vi "Test MultiValue INSERT.vi"() -> ()   [LabVIEW 2013, in "PQ Connection.lvclass"]
uses:
  Connection/PQ Connection.lvclass
  Result/PQ Result.lvclass/PQ Result.ctl
  Connection/Execute Command (No results).vi
  Result/Clear.vi
  Connection/Execute Command (Result).vi
  Connection/Execute (no results).vi
  Connection/Execute (Return first result with rows).vi
  Connection/Single Command with parameters.vi
  1. Sources/Lib/Lib.llb/Trim Whitespace (String)__ogtk.vi
panel:
  in  "Old":bool
  out "concatenated string":string
  in  "Connection Strings to access PostgreSQL":string="host=localhost port=5432 dbname = mydb "
  out "INSERTS/sec":dbl format="%#_3p"
  out "Time per INSERT":dbl format="%#_3p"
  out "error out":errorcluster
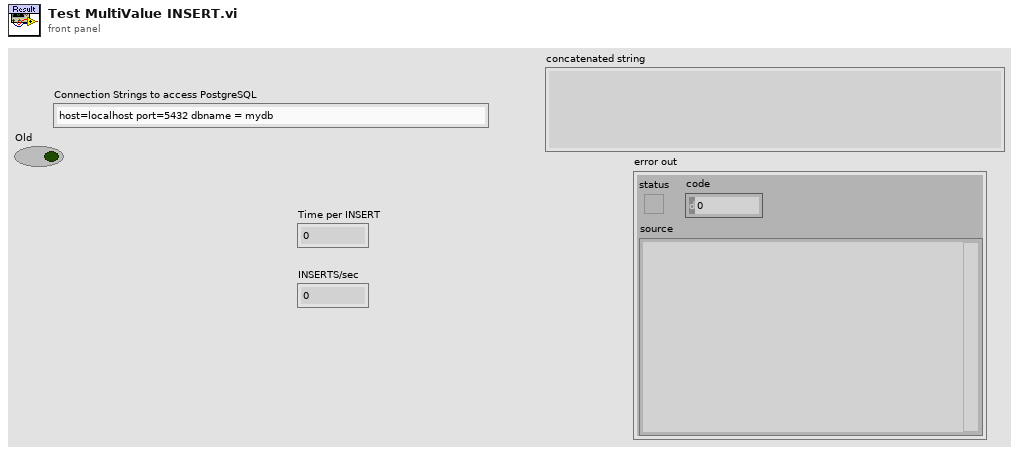
[diagram p1: front panel]
types:
  T1 = cluster{i32, "number: 0 to 1":dbl, string, "seconds since 1Jan1904":timestamp}
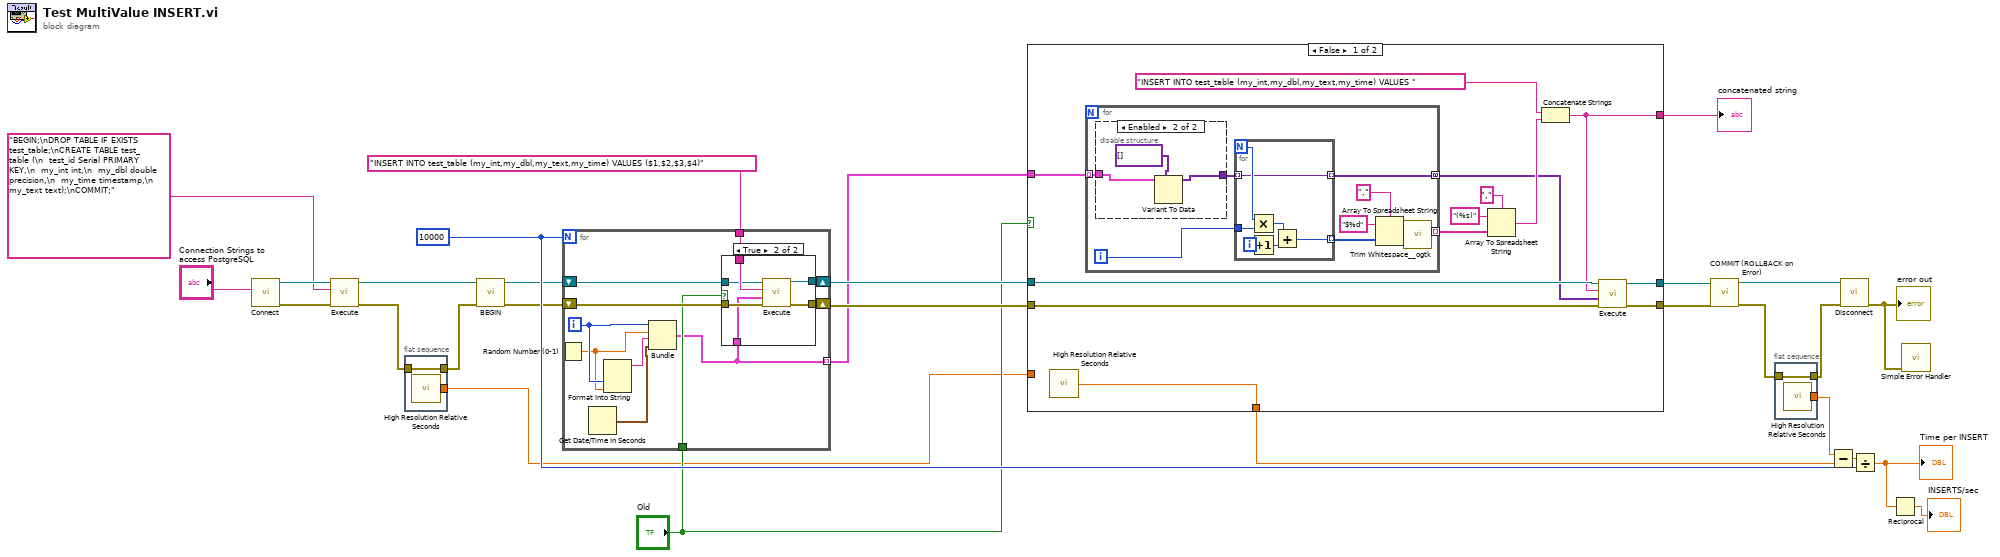
[diagram p0: block diagram]
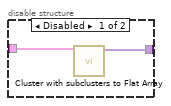
[diagram p2: hidden frame]
diagram:
  w15 = 10000
  n1 = call "Connect.vi"("Connection Strings"="Connection Strings to access PostgreSQL") -> ("error out"=w23:errorcluster, "PQ Connection out"=w25:refnum<class "PQ Connection.lvclass">)  [unwired: 9 in]
  n2 = call-poly "Execute.vi"("error in (no error)"=w23, "SQL"="BEGIN;\nDROP TABLE IF EXISTS test_table;\nCREATE TABLE test_table (\n  test_id Serial PRIMARY KEY,\n  my_int int,\n  my_dbl double precision,\n  my_time timestamp,\n  my_text text);\nCOMMIT;", "PQ Connection in"=w25) -> ("error out"=w20:errorcluster, "PQ Connection out"=w24:refnum<class "PQ Connection.lvclass">)  [unwired: 7 in]
  n3 = flat-sequence {
    tunnel: w20 -> [w30]
    tunnel: [w30] -> w13
    tunnel: [w29] -> w2
    frame #0 {
      n4 = call <vilib>:"High Resolution Relative Seconds.vi"() -> ("relative seconds"=w29:dbl)
    }
  }
  n5 = call "BEGIN.vi"("error in (no error)"=w13, "PQ Connection in"=w24) -> ("error out"=w12:errorcluster, "PQ Connection out"=w14:refnum<class "PQ Connection.lvclass">)  [unwired: 8 in]
  n6 = for {
    N: w15 -> [_]
    tunnel: "INSERT INTO test_table (my_int,my_dbl,my_text,my_time) VALUES ($1,$2,$3,$4)" ("command") -> [w40]
    shift-right: [w41] -> w9
    shift-left: w14 -> [w39]
    shift-right: [w37] -> w6
    shift-left: w12 -> [w38]
    tunnel: [w31] -> w3 mode=indexing
    tunnel: "Old" -> [w33]
    i -> [w36]
    n7 = Random Number (0-1)() -> (number: 0 to 1=w35:dbl)
    n8 = Get Date/Time In Seconds() -> (seconds since 1Jan1904=w32:timestamp)
    n9 = Format Into String(w36, w35) -> (resulting string=w34:string)  [unwired: 3 in, 1 out]
    n10 = Bundle(w36, "number: 0 to 1"=w35, w34, "seconds since 1Jan1904"=w32) -> (w31:T1)  [unwired: 1 in]
    n11 = case shown="True" w33 {
      tunnel: [w43 w49] -> w41
      tunnel: w40 -> [_ w48]
      tunnel: w39 -> [w43 w47]
      tunnel: w38 -> [w42 w46]
      tunnel: [w42 w45] -> w37
      tunnel: w31 -> [_ w44]
      frame False {
      }
      frame True {
        n12 = call-poly "Execute.vi"("error in (no error)"=w46, "Parameters"=w44, "SQL"=w48, "PQ Connection in"=w47) -> ("error out"=w45:errorcluster, "PQ Connection out"=w49:refnum<class "PQ Connection.lvclass">)  [unwired: 6 in]
      }
    }
  }
  n13 = case shown="False" "Old" {
    tunnel: w3 -> [w62 _]
    tunnel: w9 -> [w56 w86]
    tunnel: [w55 w86] -> w8
    tunnel: [w54 w85] -> w7
    tunnel: w6 -> [w53 w85]
    tunnel: [w52 _] -> w5
    tunnel: w2 -> [_ w84]
    tunnel: [w50 w84] -> w1
    frame False {
      n14 = call <vilib>:"High Resolution Relative Seconds.vi"() -> ("relative seconds"=w50:dbl)
      n15 = for {
        tunnel: w62 -> [w71] mode=indexing
        tunnel: [w63] -> w59 mode=indexing
        tunnel: [w64] -> w51 mode=concatenating
        i -> [w69]
        n16 = disable-structure shown="Enabled" {
          disable-tunnel: w71 -> [w73 w75]
          disable-tunnel: [w72 w74] -> w70
          frame Disabled {
            n17 = call "Cluster with subclusters to Flat Array.vi"("Variant"=w73) -> ("Array of items"=w72:variant[])  [unwired: 8 in, 2 out]
          }
          frame Enabled {
            n18 = Variant To Data(type=variant[] [], Variant=w75) -> (data=w74:variant[])  [unwired: 1 in, 1 out]
          }
        }
        n19 = for {
          N -> [w82]
          tunnel: w70 -> [w78] mode=indexing
          tunnel: w69 -> [w81]
          tunnel: [w79] -> w68 mode=indexing
          tunnel: [w78] -> w64 mode=indexing
          i -> [w83]
          n20 = Multiply(x=w82, y=w81) -> (x*y=w80:i32)
          n21 = Increment(x=w83) -> (x+1=w77:i32)
          n22 = Add(x=w80, y=w77) -> (x+y=w79:i32)
        }
        n23 = Array To Spreadsheet String(delimiter (Tab)=",", array=w68, 3:"$%d" ("format string")) -> (spreadsheet string=w65:string)
        n24 = call-poly <userlib>:"Trim Whitespace__ogtk.vi"("String in"=w65) -> ("String out"=w63:string)  [unwired: 6 in]
      }
      n25 = Array To Spreadsheet String(delimiter (Tab)=",", array=w59, 3:"(%s)" ("format string")) -> (spreadsheet string=w57:string)
      n26 = Concatenate Strings("INSERT INTO test_table (my_int,my_dbl,my_text,my_time) VALUES " ("command"), w57) -> (w52:string)
      n27 = call-poly "Execute.vi"("error in (no error)"=w53, "Parameters"=w51, "SQL"=w52, "PQ Connection in"=w56) -> ("error out"=w54:errorcluster, "PQ Connection out"=w55:refnum<class "PQ Connection.lvclass">)  [unwired: 6 in]
    }
    frame True {
    }
  }
  "concatenated string" <- w5
  n28 = call "COMMIT (ROLLBACK on Error).vi"("error in (no error)"=w7, "PQ Connection in"=w8) -> ("error out"=w19:errorcluster, "PQ Connection out"=w21:refnum<class "PQ Connection.lvclass">)  [unwired: 8 in]
  n29 = flat-sequence {
    tunnel: w19 -> [w88]
    tunnel: [w88] -> w18
    tunnel: [w87] -> w17
    frame #0 {
      n30 = call <vilib>:"High Resolution Relative Seconds.vi"() -> ("relative seconds"=w87:dbl)
    }
  }
  n31 = Subtract(x=w17, y=w1) -> (x-y=w16:dbl)
  n32 = call-dynamic "Disconnect.vi"("error in (no error)"=w18, "PQ Connection in"=w21) -> ("error out"=w26:errorcluster)  [unwired: 9 in]
  "error out" <- w26
  n33 = Divide(x=w16, y=w15) -> (x/y=w11:dbl)
  "Time per INSERT" <- w11
  n34 = Reciprocal(x=w11) -> (1/x=→"INSERTS/sec":dbl)
  n35 = call <vilib>:"Simple Error Handler.vi"("error in (no error)"=w26) -> ()  [unwired: 4 in, 5 out]
